vi "Charge Pump Array to Register to Write Array.vi"(8 "error in (no error)":errorcluster, 11 "Toggle 6 in":refnum<class "Toggle 7.1.lvclass">) -> (0 "error out":errorcluster, 1 "Charge Pump Values":dbl[](array[numeric]), 2 "Charge Pump Settings":T1[](array[typedef]), 3 "Toggle 6 out":refnum<class "Toggle 7.1.lvclass">)   [LabVIEW 2020, in "Toggle 7.1.lvclass"]
doc: "Getting the Charge pump array and makes it into registers"
uses:
  Toggle 7.1.lvclass
  Controls/Register to Write.ctl
  PIC-device/PIC-Device.lvclass
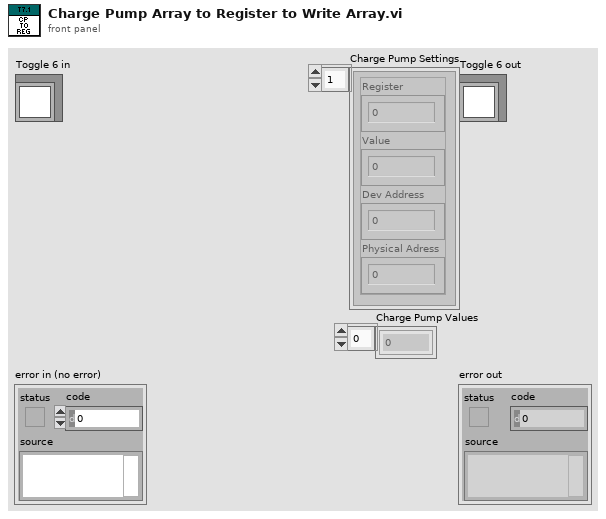
[diagram p1: front panel]
types:
  T1 = typedef "PIC-Device.lvclass/Register to Write.ctl" = cluster{"Register":u32, "Value":u32, "Dev Address":u32, "Physical Adress":u32}
  T2 = typedef "Toggle 7.1.lvclass/Parameter Cluster.ctl" = cluster{"Enable":bool, "Register Number":u32, "Use Array":bool, "Array":dbl[], "To From Cluster":cluster{"From":dbl, "To":dbl, "Step":dbl}}
  T3 = typedef "Toggle 7.1.lvclass/Charge Pump Information cluster.ctl" = cluster{"Min":dbl, "Max":dbl, "Step":dbl, "Default":dbl}
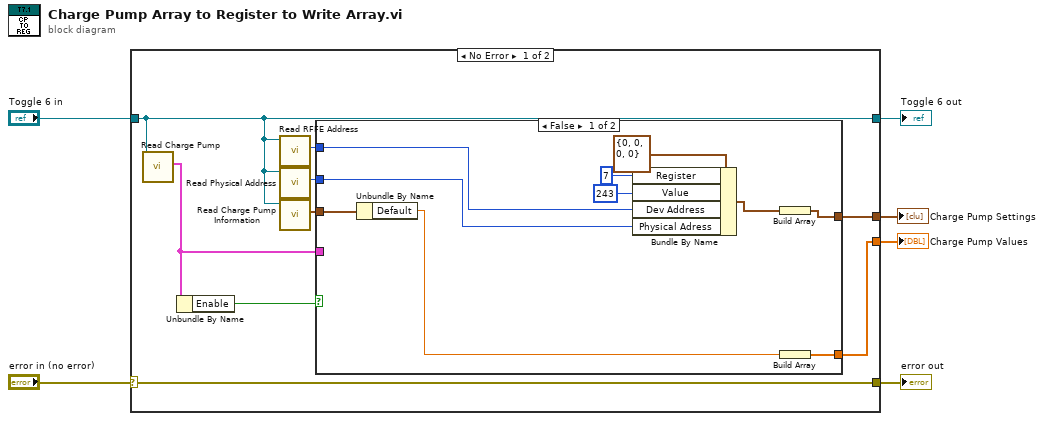
[diagram p0: block diagram]
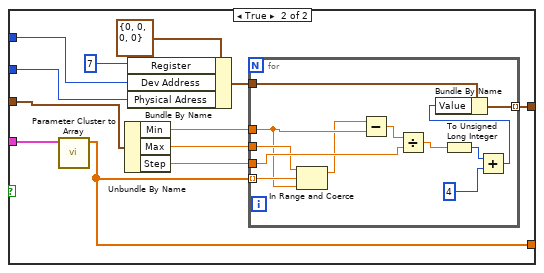
[diagram p2: hidden frame]
diagram:
  n1 = case shown="No Error" "error in (no error)" {
    selector: "error in (no error)" -> [w15 w51]
    tunnel: [w15 w51] -> w5
    tunnel: [w13 w50] -> w3
    tunnel: "Toggle 6 in" -> [w13 w50]
    tunnel: [w14 _] -> w2
    tunnel: [w11 _] -> w1
    frame No Error {
      n2 = call-dynamic "Read Charge Pump.vi"("Toggle 7.1 in"=w13) -> ("Parameter Cluster"=w12:T2)  [unwired: 8 in, 2 out]
      n3 = Unbundle By Name(w12) -> ("Enable"=w7:bool)
      n4 = call-dynamic "Read RFFE Address.vi"("Toggle 6 in"=w13) -> ("RFFE Adress"=w10:u32)  [unwired: 8 in, 2 out]
      n5 = call-dynamic "Read Physical Address.vi"("Toggle 6 in"=w13) -> ("Physical Adress"=w9:u32)  [unwired: 9 in, 1 out]
      n6 = call-dynamic "Read Charge Pump Information.vi"("Toggle 6 in"=w13) -> ("Charge Pump Information"=w8:T3)  [unwired: 9 in, 1 out]
      n7 = case shown="False" w7 {
        tunnel: [w16 w37] -> w14
        tunnel: w12 -> [_ w36]
        tunnel: [w24 w35] -> w11
        tunnel: w10 -> [w19 w32]
        tunnel: w9 -> [w18 w31]
        tunnel: w8 -> [w25 w29]
        frame False {
          n8 = Unbundle By Name(w25) -> ("Default"=w23:dbl)
          n9 = Bundle By Name(cluster=T1 {"Register"=0, "Value"=0, "Dev Address"=0, "Physical Adress"=0} ("Register to Write"), "Register"=u32 7, "Value"=u32 243, "Dev Address"=w19, "Physical Adress"=w18) -> (w17:T1)
          n10 = Build Array(w17) -> (w16:T1[])
          n11 = Build Array(w23) -> (w24:dbl[])
        }
        frame True {
          n12 = call "Parameter Cluster to Array.vi"("Parameter Cluster"=w36) -> ("Array"=w35:dbl[])  [unwired: 10 in]
          n13 = Unbundle By Name(w29) -> ("Min"=w28:dbl, "Max"=w27:dbl, "Step"=w26:dbl)
          n14 = Bundle By Name(cluster=T1 {"Register"=0, "Value"=0, "Dev Address"=0, "Physical Adress"=0} ("Register to Write"), "Register"=u32 7, "Dev Address"=w32, "Physical Adress"=w31) -> (w30:T1)
          n15 = for {
            tunnel: w30 -> [w49]
            tunnel: w35 -> [w46] mode=indexing
            tunnel: w28 -> [w44]
            tunnel: w27 -> [w45]
            tunnel: w26 -> [w47]
            tunnel: [w41] -> w37 mode=indexing
            n16 = In Range and Coerce(upper limit=w45, x=w46, lower limit=w44) -> (coerced(x)=w43:dbl)  [unwired: 1 out]
            n17 = Subtract(x=w43, y=w44) -> (x-y=w48:dbl)
            n18 = Divide(x=w48, y=w47) -> (x/y=w42:dbl)
            n19 = To Unsigned Long Integer(number=w42) -> (unsigned 32bit integer=w40:u32)
            n20 = Add(x=w40, y=u32 4 ("unsigned 32bit integer")) -> (x+y=w38:u32)
            n21 = Bundle By Name(cluster=w49, "Value"=w38) -> (w41:T1)
          }
        }
      }
    }
    frame Error {
    }
  }
  "error out" <- w5
  "Toggle 6 out" <- w3
  "Charge Pump Settings" <- w2
  "Charge Pump Values" <- w1
